vi "Parse Label.vi"(0 "Stage Controller in":refnum<class "Stage Controller.lvclass">, 5 "Label.Text":string, 11 "error in (no error)":errorcluster) -> (4 "Stage Controller out":refnum<class "Stage Controller.lvclass">, 6 "Stage Label":string, 8 "Increase?":bool=TRUE, 10 "Big Step?":bool, 15 "error out":errorcluster)   [LabVIEW 2020, in "Stage.lvlib" / "Stage Controller.lvlib" / "Stage Controller.lvclass"]
uses:
  Stage Controller.lvclass
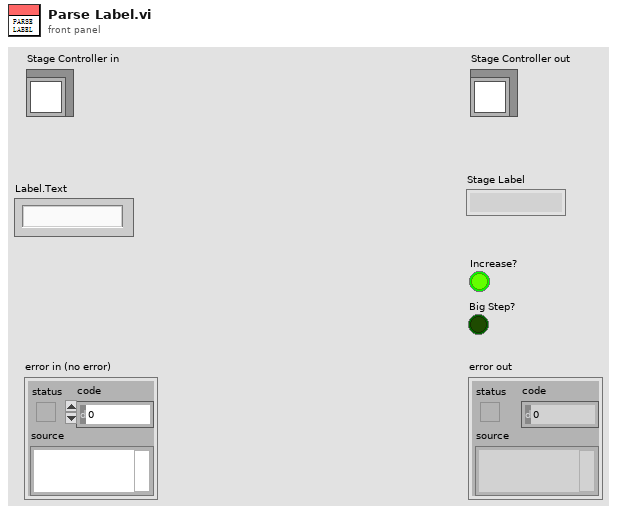
[diagram p1: front panel]
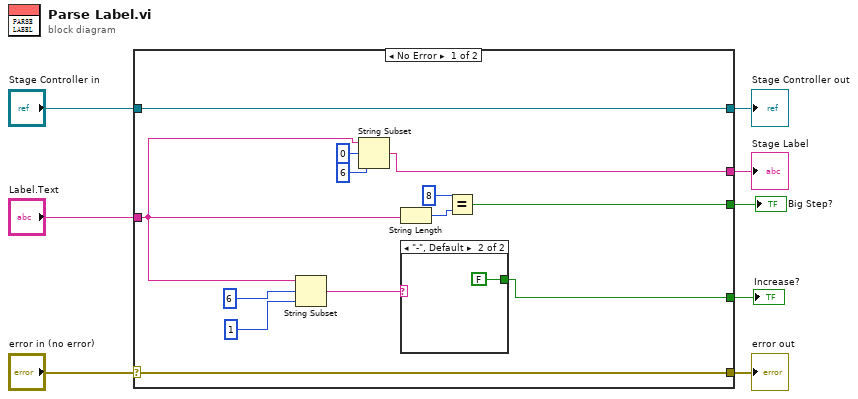
[diagram p0: block diagram]
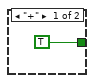
[diagram p2: hidden frame]
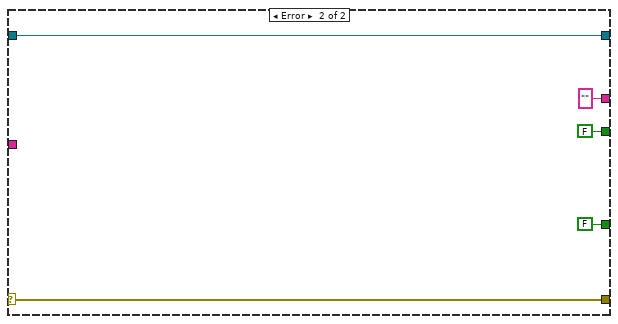
[diagram p3: hidden frame]
diagram:
  n1 = case shown="No Error" "error in (no error)" {
    selector: "error in (no error)" -> [w20 w28]
    tunnel: [w20 w28] -> w7
    tunnel: [w21 w27] -> w5
    tunnel: "Stage Controller in" -> [w21 w27]
    tunnel: "Label.Text" -> [w13 _]
    tunnel: [w12 FALSE] -> w3
    tunnel: [w11 "" ("Label.Text")] -> w2
    tunnel: [w10 FALSE ("Increase?")] -> w1
    frame No Error {
      n2 = String Subset(string=w13, offset (0)=6, length (rest)=1 ("length (rest)")) -> (substring=w9:string)
      n3 = String Subset(string=w13, offset (0)=0, length (rest)=6 ("length (rest)")) -> (substring=w11:string)
      n4 = String Length(string=w13) -> (length=w15:i32)
      n5 = case shown="\"-\", Default" w9 {
        tunnel: [TRUE ("Increase?") FALSE ("Increase?")] -> w10
        frame "+" {
        }
        frame "-", Default {
        }
      }
      n6 = Equal?(x=8, y=w15) -> (x = y?=w12:bool)
    }
    frame Error {
    }
  }
  "error out" <- w7
  "Stage Controller out" <- w5
  "Increase?" <- w1
  "Stage Label" <- w2
  "Big Step?" <- w3
